vi "old_FSM.vi"() -> ()   [LabVIEW 2015]
uses:
  states.ctl
  globals.vi
  <vilib>/Utility/file.llb/Read Delimited Spreadsheet (DBL).vi
  read_file.vi
  output_byte.vi
panel:
  out "Progress":dbl(slide) scale=0.0..100.0
  out "Angle accuracy":dbl
  in  "Input file":path
  out "Current shoulder angle":dbl
  out "Current elbow angle":dbl
  in  "Stop":bool
  out "Desired shoulder Angle":dbl
  out "Desired elbow Angle":dbl
  out "Number of rows":dbl
  out "Row number":dbl
  in  "Start Button":bool
  out "State to Recover from":T1
  out "Current State":T1
  in  "Pause":bool
  # ".csv file with contours"
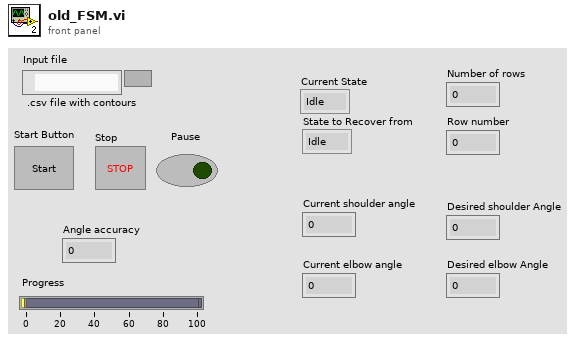
[diagram p1: front panel]
types:
  T1 = typedef "states.ctl" = enum16{"Idle", "Pause", "Next Contour", "Aligning", "Lowering Pen", "Drawing", "Next Point", "Lifting Pen", "Stop", "Put Away"}
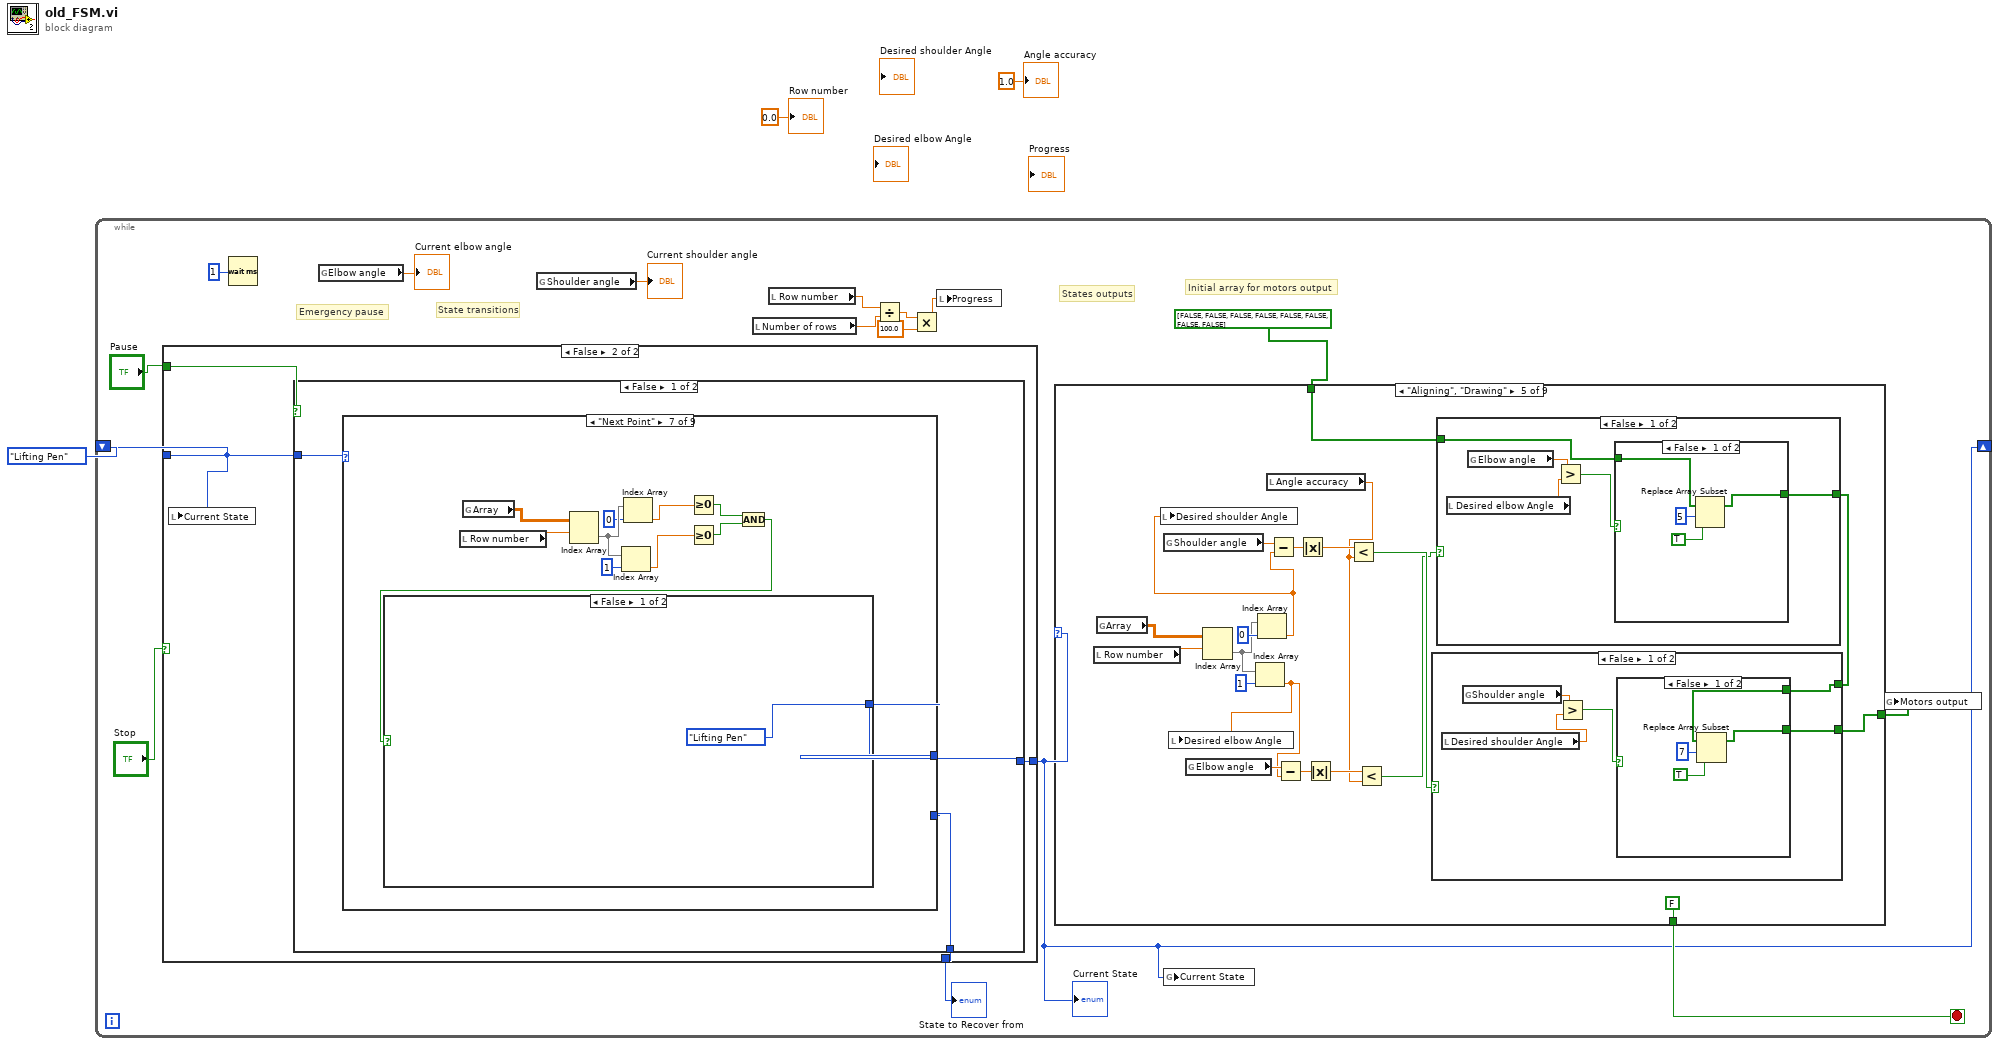
[diagram p0: block diagram]
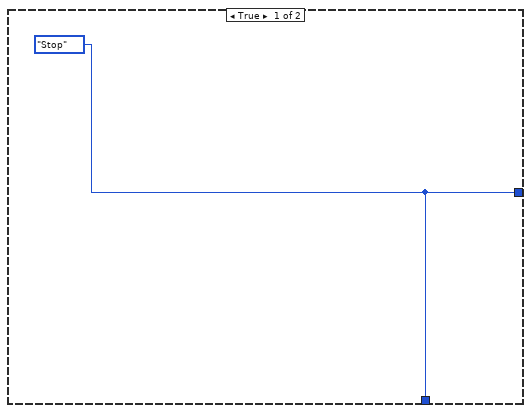
[diagram p2: hidden frame]
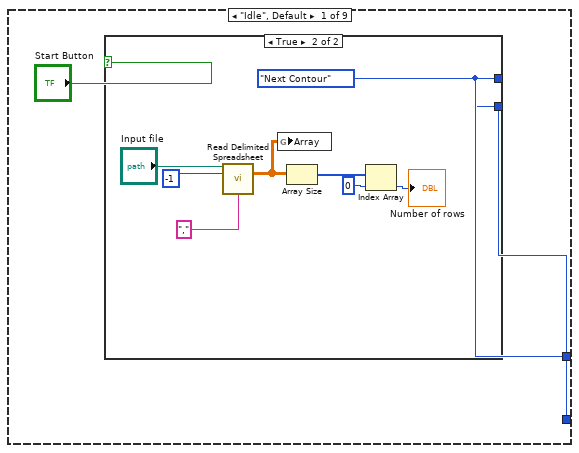
[diagram p3: hidden frame]
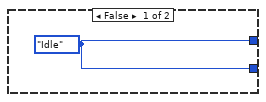
[diagram p4: hidden frame]
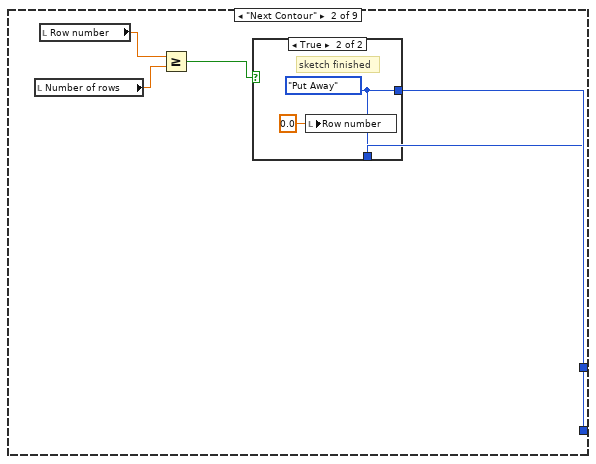
[diagram p5: hidden frame]
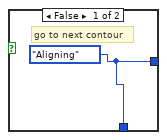
[diagram p6: hidden frame]
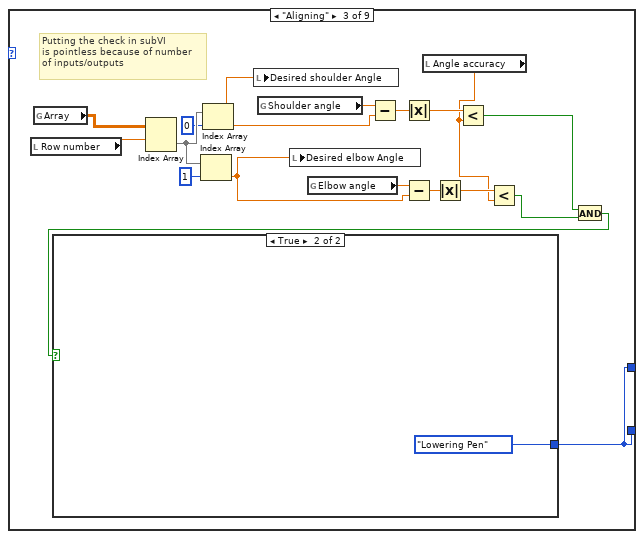
[diagram p7: hidden frame]
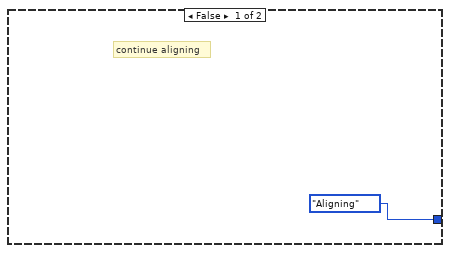
[diagram p8: hidden frame]
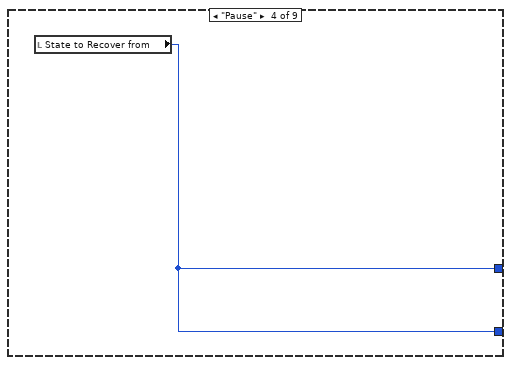
[diagram p9: hidden frame]
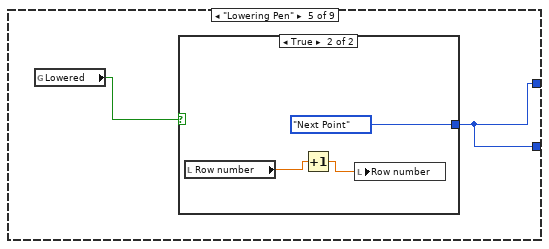
[diagram p10: hidden frame]
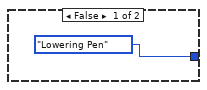
[diagram p11: hidden frame]
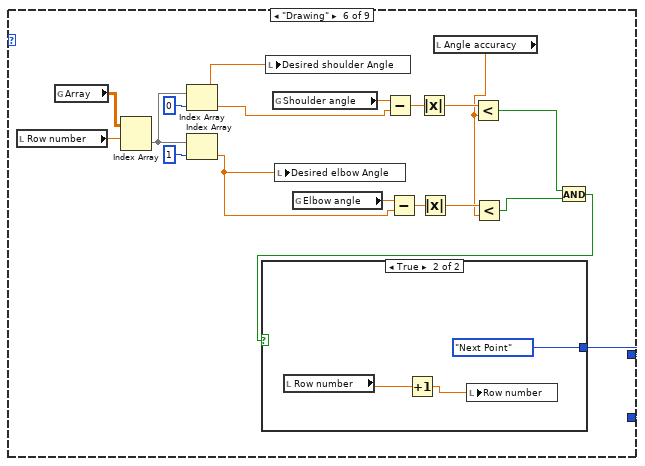
[diagram p12: hidden frame]
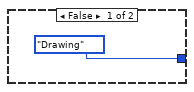
[diagram p13: hidden frame]
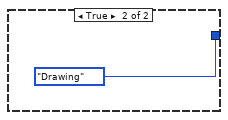
[diagram p14: hidden frame]
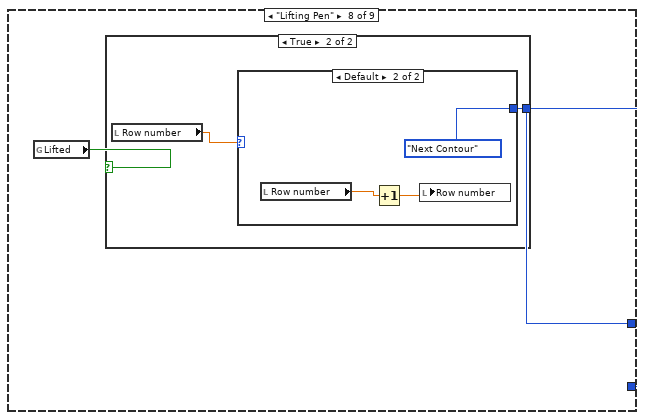
[diagram p15: hidden frame]
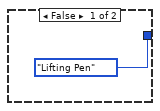
[diagram p16: hidden frame]
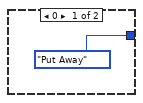
[diagram p17: hidden frame]
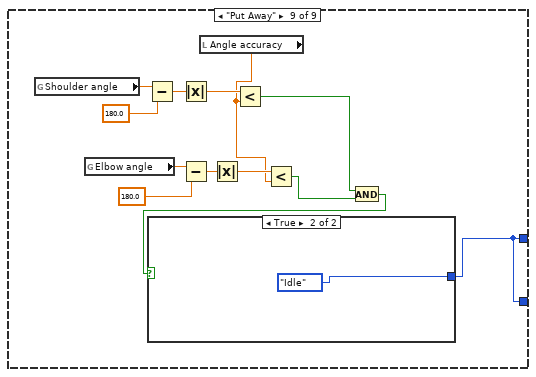
[diagram p18: hidden frame]
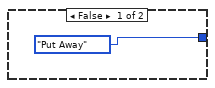
[diagram p19: hidden frame]
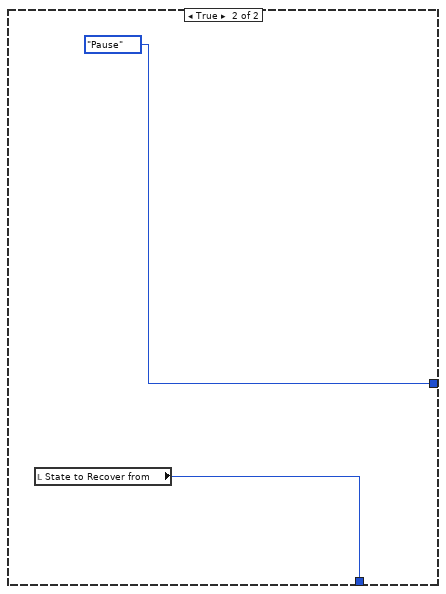
[diagram p20: hidden frame]
diagram:
  n1 = while {
    shift-right: [w4] -> _
    shift-left: states."Lifting Pen" ("State") -> [w18]
    stop <- w5 stop-if-true
    # "Initial array for motors output"
    # "States outputs"
    # "State transitions"
    # "Emergency pause"
    n2 = case shown="False" "Stop" {
      tunnel: "Pause" -> [_ w24]
      tunnel: w18 -> [_ w23]
      tunnel: [w20 w22] -> w14
      tunnel: [w20 w21] -> w4
      frame True {
        w20 = states."Stop" ("State")
      }
      frame False {
        n3 = local write "Current State"(w23) -> ()
        n4 = case shown="False" w24 {
          tunnel: w23 -> [w27 _]
          tunnel: [w26 states."Pause" ("State")] -> w21
          tunnel: [w25 w134] -> w22
          frame False {
            n5 = case shown="\"Next Point\"" w27 {
              tunnel: [w29 w44 w52 w68 w70 w78 w98 w111 w119] -> w26
              tunnel: [w28 w43 w52 w68 w70 w78 w98 w111 w119] -> w25
              frame "Idle", Default {
                n6 = case shown="True" "Start Button" {
                  tunnel: [w31 w39] -> w29
                  tunnel: [w31 w39] -> w28
                  frame False {
                    w31 = states."Idle" ("State")
                  }
                  frame True {
                    w39 = states."Next Contour" ("State")
                    n7 = call-poly <vilib>:"Read Delimited Spreadsheet.vi"("file path (dialog if empty)"="Input file", "number of rows (all:-1)"=-1, "delimiter (\\t)"="," ("delimiter (\\t)")) -> ("all rows"=w38:dbl[][])  [unwired: 7 in, 5 out]
                    n8 = global write "read_file.vi" "Array"(w38) -> ()
                    n9 = Array Size(array=w38) -> (size(s)=w33:i32[])
                    n10 = Index Array(array=w33, index=0) -> (element=→"Number of rows":i32)
                  }
                }
              }
              frame "Next Contour" {
                n11 = local read "Number of rows"() -> (w41:dbl)
                n12 = local read "Row number"() -> (w42:dbl)
                n13 = Greater Or Equal?(x=w42, y=w41) -> (x >= y?=w40:bool)
                n14 = case shown="True" w40 {
                  tunnel: [w45 w47] -> w44
                  tunnel: [w45 w47] -> w43
                  frame False {
                    w45 = states."Aligning" ("State")
                    # "go to next contour"
                  }
                  frame True {
                    w47 = states."Put Away" ("State")
                    # "sketch finished"
                    n15 = local write "Row number"(0.0 ("Row number")) -> ()
                  }
                }
              }
              frame "Aligning" {
                # "Putting the check in subVI\nis pointless because of number\nof inputs/outputs"
                n16 = local read "Row number"() -> (w64:dbl)
                n17 = global read "read_file.vi" "Array"() -> (w65:dbl[][])
                n18 = Index Array(array=w65, index (row)=w64) -> (element=w63:dbl[])  [unwired: 1 in]
                n19 = Index Array(array=w63, index=1) -> (element=w55:dbl)
                n20 = Index Array(array=w63, index=0) -> (element=w56:dbl)
                n21 = local write "Desired shoulder Angle"(w56) -> ()
                n22 = global read "globals.vi" "Shoulder angle"() -> (w51:dbl)
                n23 = local write "Desired elbow Angle"(w55) -> ()
                n24 = global read "globals.vi" "Elbow angle"() -> (w50:dbl)
                n25 = Subtract(x=w51, y=w56) -> (x-y=w60:dbl)
                n26 = Absolute Value(x=w60) -> (abs(x)=w59:dbl)
                n27 = Subtract(x=w50, y=w55) -> (x-y=w58:dbl)
                n28 = local read "Angle accuracy"() -> (w48:dbl)
                n29 = Absolute Value(x=w58) -> (abs(x)=w57:dbl)
                n30 = Less?(x=w59, y=w48) -> (x < y?=w54:bool)
                n31 = Less?(x=w57, y=w48) -> (x < y?=w53:bool)
                n32 = And(x=w54, y=w53) -> (x .and. y?=w49:bool)
                n33 = case shown="True" w49 {
                  tunnel: [states."Aligning" ("State") states."Lowering Pen" ("State")] -> w52
                  frame False {
                    # "continue aligning"
                  }
                  frame True {
                  }
                }
              }
              frame "Pause" {
                n34 = local read "State to Recover from"() -> (w68:T1)
              }
              frame "Lowering Pen" {
                n35 = global read "globals.vi" "Lowered"() -> (w69:bool)
                n36 = case shown="True" w69 {
                  tunnel: [states."Lowering Pen" ("State") states."Next Point" ("State")] -> w70
                  frame False {
                  }
                  frame True {
                    n37 = local read "Row number"() -> (w72:dbl)
                    n38 = Increment(x=w72) -> (x+1=w73:dbl)
                    n39 = local write "Row number"(w73) -> ()
                  }
                }
              }
              frame "Drawing" {
                n40 = local read "Row number"() -> (w79:dbl)
                n41 = global read "read_file.vi" "Array"() -> (w92:dbl[][])
                n42 = Index Array(array=w92, index (row)=w79) -> (element=w91:dbl[])  [unwired: 1 in]
                n43 = Index Array(array=w91, index=0) -> (element=w77:dbl)
                n44 = Index Array(array=w91, index=1) -> (element=w84:dbl)
                n45 = local write "Desired shoulder Angle"(w77) -> ()
                n46 = global read "globals.vi" "Shoulder angle"() -> (w81:dbl)
                n47 = local write "Desired elbow Angle"(w84) -> ()
                n48 = global read "globals.vi" "Elbow angle"() -> (w80:dbl)
                n49 = Subtract(x=w81, y=w77) -> (x-y=w88:dbl)
                n50 = Subtract(x=w80, y=w84) -> (x-y=w86:dbl)
                n51 = Absolute Value(x=w88) -> (abs(x)=w87:dbl)
                n52 = Absolute Value(x=w86) -> (abs(x)=w85:dbl)
                n53 = local read "Angle accuracy"() -> (w75:dbl)
                n54 = Less?(x=w87, y=w75) -> (x < y?=w83:bool)
                n55 = Less?(x=w85, y=w75) -> (x < y?=w82:bool)
                n56 = And(x=w83, y=w82) -> (x .and. y?=w76:bool)
                n57 = case shown="True" w76 {
                  tunnel: [states."Drawing" ("State") states."Next Point" ("State")] -> w78
                  frame False {
                  }
                  frame True {
                    n58 = local read "Row number"() -> (w95:dbl)
                    n59 = Increment(x=w95) -> (x+1=w94:dbl)
                    n60 = local write "Row number"(w94) -> ()
                  }
                }
              }
              frame "Next Point" {
                n61 = local read "Row number"() -> (w106:dbl)
                n62 = global read "read_file.vi" "Array"() -> (w107:dbl[][])
                n63 = Index Array(array=w107, index (row)=w106) -> (element=w105:dbl[])  [unwired: 1 in]
                n64 = Index Array(array=w105, index=1) -> (element=w101:dbl)
                n65 = Index Array(array=w105, index=0) -> (element=w102:dbl)
                n66 = Greater Or Equal To 0?(x=w102) -> (x >= 0?=w100:bool)
                n67 = Greater Or Equal To 0?(x=w101) -> (x >= 0?=w99:bool)
                n68 = And(x=w100, y=w99) -> (x .and. y?=w97:bool)
                n69 = case shown="False" w97 {
                  tunnel: [states."Lifting Pen" ("State") states."Drawing" ("State")] -> w98
                  frame False {
                  }
                  frame True {
                  }
                }
              }
              frame "Lifting Pen" {
                n70 = global read "globals.vi" "Lifted"() -> (w110:bool)
                n71 = case shown="True" w110 {
                  tunnel: [states."Lifting Pen" ("State") w114] -> w111
                  frame False {
                  }
                  frame True {
                    n72 = local read "Row number"() -> (w113:dbl)
                    n73 = case shown="Default" w113 {
                      tunnel: [states."Put Away" ("State") states."Next Contour" ("State")] -> w114
                      frame 0 {
                      }
                      frame Default {
                        n74 = local read "Row number"() -> (w117:dbl)
                        n75 = Increment(x=w117) -> (x+1=w116:dbl)
                        n76 = local write "Row number"(w116) -> ()
                      }
                    }
                  }
                }
              }
              frame "Put Away" {
                n77 = global read "globals.vi" "Shoulder angle"() -> (w125:dbl)
                n78 = global read "globals.vi" "Elbow angle"() -> (w124:dbl)
                n79 = Subtract(x=w125, y=180.0) -> (x-y=w131:dbl)
                n80 = Absolute Value(x=w131) -> (abs(x)=w130:dbl)
                n81 = Subtract(x=w124, y=180.0) -> (x-y=w129:dbl)
                n82 = local read "Angle accuracy"() -> (w123:dbl)
                n83 = Absolute Value(x=w129) -> (abs(x)=w128:dbl)
                n84 = Less?(x=w130, y=w123) -> (x < y?=w127:bool)
                n85 = Less?(x=w128, y=w123) -> (x < y?=w126:bool)
                n86 = And(x=w127, y=w126) -> (x .and. y?=w120:bool)
                n87 = case shown="True" w120 {
                  tunnel: [states."Put Away" ("State") states."Idle" ("State")] -> w119
                  frame False {
                  }
                  frame True {
                  }
                }
              }
            }
          }
          frame True {
            n88 = local read "State to Recover from"() -> (w134:T1)
          }
        }
      }
    }
    "Current State" <- w4
    "State to Recover from" <- w14
    n89 = Wait (ms)(milliseconds to wait=u32 1 ("millisecond multiple")) -> ()  [unwired: 1 out]
    n90 = global read "globals.vi" "Elbow angle"() -> (→"Current elbow angle":dbl)
    n91 = global read "globals.vi" "Shoulder angle"() -> (→"Current shoulder angle":dbl)
    n92 = local read "Number of rows"() -> (w10:dbl)
    n93 = local read "Row number"() -> (w11:dbl)
    n94 = Divide(x=w11, y=w10) -> (x/y=w9:dbl)
    n95 = Multiply(x=w9, y=100.0) -> (x*y=w7:dbl)
    n96 = local write "Progress"(w7) -> ()
    n97 = case shown="\"Aligning\", \"Drawing\"" w4 {
      tunnel: bool[] [FALSE, FALSE, FALSE, FALSE, FALSE, FALSE, FALSE, FALSE] -> [w137 w139 w141 w144 w165 w196 w199 w203 w207]
      tunnel: [w137 w139 w141 w143 w164 w196 w198 w203 w204] -> w12
      tunnel: [FALSE FALSE FALSE FALSE FALSE FALSE FALSE TRUE FALSE] -> w5
      frame "Idle", Default {
      }
      frame "Pause" {
      }
      frame "Next Contour" {
      }
      frame "Lowering Pen" {
        n98 = Replace Array Subset(array=w144, new element=TRUE ("new element/subarray"), index=2) -> (w143:bool[])
      }
      frame "Aligning", "Drawing" {
        n99 = local read "Row number"() -> (w160:dbl)
        n100 = global read "read_file.vi" "Array"() -> (w159:dbl[][])
        n101 = global read "globals.vi" "Shoulder angle"() -> (w158:dbl)
        n102 = global read "globals.vi" "Elbow angle"() -> (w154:dbl)
        n103 = Index Array(array=w159, index (row)=w160) -> (element=w161:dbl[])  [unwired: 1 in]
        n104 = Index Array(array=w161, index=1) -> (element=w151:dbl)
        n105 = local write "Desired elbow Angle"(w151) -> ()
        n106 = Index Array(array=w161, index=0) -> (element=w155:dbl)
        n107 = local write "Desired shoulder Angle"(w155) -> ()
        n108 = local read "Angle accuracy"() -> (w148:dbl)
        n109 = Subtract(x=w158, y=w155) -> (x-y=w156:dbl)
        n110 = Subtract(x=w154, y=w151) -> (x-y=w152:dbl)
        n111 = Absolute Value(x=w156) -> (abs(x)=w157:dbl)
        n112 = Absolute Value(x=w152) -> (abs(x)=w153:dbl)
        n113 = Less?(x=w157, y=w148) -> (x < y?=w150:bool)
        n114 = Less?(x=w153, y=w148) -> (x < y?=w149:bool)
        n115 = case shown="False" w149 {
          tunnel: [w182 w194] -> w166
          tunnel: w165 -> [w181 w194]
          frame False {
            n116 = local read "Desired elbow Angle"() -> (w185:dbl)
            n117 = global read "globals.vi" "Elbow angle"() -> (w183:dbl)
            n118 = Greater?(x=w183, y=w185) -> (0:w184:bool)
            n119 = case shown="False" w184 {
              tunnel: [w187 w191] -> w182
              tunnel: w181 -> [w186 w190]
              frame False {
                n120 = Replace Array Subset(array=w186, new element=TRUE ("new element/subarray"), index=5) -> (w187:bool[])
              }
              frame True {
                n121 = Replace Array Subset(array=w190, new element=TRUE ("new element/subarray"), index=4) -> (w191:bool[])
              }
            }
          }
          frame True {
          }
        }
        n122 = case shown="False" w150 {
          tunnel: [w169 w180] -> w164
          tunnel: w166 -> [w167 w180]
          frame False {
            n123 = local read "Desired shoulder Angle"() -> (w168:dbl)
            n124 = global read "globals.vi" "Shoulder angle"() -> (w170:dbl)
            n125 = Greater?(x=w170, y=w168) -> (0:w171:bool)
            n126 = case shown="False" w171 {
              tunnel: [w173 w177] -> w169
              tunnel: w167 -> [w172 w176]
              frame False {
                n127 = Replace Array Subset(array=w172, new element=TRUE ("new element/subarray"), index=7) -> (w173:bool[])
              }
              frame True {
                n128 = Replace Array Subset(array=w176, new element=TRUE ("new element/subarray"), index=6) -> (w177:bool[])
              }
            }
          }
          frame True {
          }
        }
      }
      frame "Next Point" {
      }
      frame "Lifting Pen" {
        n129 = Replace Array Subset(array=w199, new element=TRUE ("new element/subarray"), index=3) -> (w198:bool[])
      }
      frame "Stop" {
      }
      frame "Put Away" {
        n130 = global read "globals.vi" "Shoulder angle"() -> (w216:dbl)
        n131 = global read "globals.vi" "Elbow angle"() -> (w213:dbl)
        n132 = local read "Angle accuracy"() -> (w208:dbl)
        n133 = Subtract(x=w216, y=180.0) -> (x-y=w214:dbl)
        n134 = Subtract(x=w213, y=180.0) -> (x-y=w211:dbl)
        n135 = Absolute Value(x=w214) -> (abs(x)=w215:dbl)
        n136 = Absolute Value(x=w211) -> (abs(x)=w212:dbl)
        n137 = Less?(x=w215, y=w208) -> (x < y?=w210:bool)
        n138 = Less?(x=w212, y=w208) -> (x < y?=w209:bool)
        n139 = case shown="False" w209 {
          tunnel: [w235 w246] -> w217
          tunnel: w207 -> [w234 w246]
          frame False {
            n140 = global read "globals.vi" "Elbow angle"() -> (w236:dbl)
            n141 = Greater?(x=w236, y=180.0) -> (0:w237:bool)
            n142 = case shown="False" w237 {
              tunnel: [w239 w243] -> w235
              tunnel: w234 -> [w238 w242]
              frame False {
                n143 = Replace Array Subset(array=w238, new element=TRUE ("new element/subarray"), index=5) -> (w239:bool[])
              }
              frame True {
                n144 = Replace Array Subset(array=w242, new element=TRUE ("new element/subarray"), index=4) -> (w243:bool[])
              }
            }
          }
          frame True {
          }
        }
        n145 = case shown="False" w210 {
          tunnel: [w221 w232] -> w204
          tunnel: w217 -> [w220 w232]
          frame False {
            n146 = global read "globals.vi" "Shoulder angle"() -> (w222:dbl)
            n147 = Greater?(x=w222, y=180.0) -> (0:w223:bool)
            n148 = case shown="False" w223 {
              tunnel: [w225 w229] -> w221
              tunnel: w220 -> [w224 w228]
              frame False {
                n149 = Replace Array Subset(array=w224, new element=TRUE ("new element/subarray"), index=7) -> (w225:bool[])
              }
              frame True {
                n150 = Replace Array Subset(array=w228, new element=TRUE ("new element/subarray"), index=6) -> (w229:bool[])
              }
            }
          }
          frame True {
          }
        }
      }
    }
    n151 = global write "output_byte.vi" "Current State"(w4) -> ()
    n152 = global write "output_byte.vi" "Motors output"(w12) -> ()
  }
  "Row number" <- 0.0 ("Row number")
  "Angle accuracy" <- 1.0 ("Angle accuracy")
